vi "TEST - Reorder Array.vi"(8 "error in (no error)":errorcluster) -> (0 "error out":errorcluster, 2 "Pass?":bool=TRUE)   [LabVIEW 2020]
doc: "This VI template can be used for the functional testing of VIs; this implementation includes handling for the testing of polymorphic VIs, and the polymorphic elements should be removed if not needed.\n\nCoded by Douglas A. Femec, January 24, 2006.\n\nCopyright (c) 2005-2006 MKS Instruments, Inc.\nAll rights reserved."
uses:
  TEST - Reorder Array - Inputs.ctl
  Polymorphizer+ Data Type.ctl
  TEST - Reorder Array - Outputs.ctl
  source/library/Reorder Array/Reorder 2D Array (EXT).vi
  source/library/Reorder Array/Reorder 1D Array (EXT).vi
  source/library/Reorder Array/Reorder 2D Array (Boolean).vi
  source/library/Reorder Array/Reorder 1D Array (Boolean).vi
  source/library/Reorder Array/Reorder 2D Array (Variant).vi
  source/library/Reorder Array/Reorder 1D Array (Variant).vi
  source/library/Reorder Array/Reorder 2D Array (DBL).vi
  source/library/Reorder Array/Reorder 1D Array (DBL).vi
  source/library/Reorder Array/Reorder 2D Array (SGL).vi
  source/library/Reorder Array/Reorder 1D Array (SGL).vi
  source/library/Reorder Array/Reorder 2D Array (I32).vi
  source/library/Reorder Array/Reorder 1D Array (I32).vi
  source/library/Reorder Array/Reorder 2D Array (I16).vi
  source/library/Reorder Array/Reorder 1D Array (I16).vi
  source/library/Reorder Array/Reorder 2D Array (I8).vi
  source/library/Reorder Array/Reorder 1D Array (I8).vi
  source/library/Reorder Array/Reorder 2D Array (U32).vi
  source/library/Reorder Array/Reorder 1D Array (U32).vi
  source/library/Reorder Array/Reorder 2D Array (U16).vi
  source/library/Reorder Array/Reorder 1D Array (U16).vi
  source/library/Reorder Array/Reorder 2D Array (U8).vi
  source/library/Reorder Array/Reorder 1D Array (U8).vi
  source/library/Reorder Array/Reorder 2D Array (CXT).vi
  source/library/Reorder Array/Reorder 1D Array (CXT).vi
  source/library/Reorder Array/Reorder 2D Array (CDB).vi
  source/library/Reorder Array/Reorder 1D Array (CDB).vi
  source/library/Reorder Array/Reorder 2D Array (CSG).vi
  source/library/Reorder Array/Reorder 1D Array (CSG).vi
  source/library/Reorder Array/Reorder 2D Array (String).vi
  source/library/Reorder Array/Reorder 1D Array (String).vi
  source/library/Reorder Array/Reorder 2D Array (Path).vi
  source/library/Reorder Array/Reorder 1D Array (Path).vi
  source/library/openg_array.lvlib
panel:
  out "Generated Outputs":T1[][](array[typedef]) {"1D Array" format="%.2f"; "2D Array" format="%.2f"}
  in  "Expected Outputs":T1[](array[typedef])=[{"Description"="Expect empty arrays", "1D Array"=[], "2D Array"=[], "1D Sorted Pointers"=[], "2D Sorted Pointer"=[], "Sort By in"=enum."row"}, {"Description"="Expect empty arrays", "1D Array"=[], "2D Array"=[], "1D Sorted Pointers"=[], "2D Sorted Pointer"=[], "Sort By in"=enum."row"}, {"Description"="Expect empty arrays", "1D Array"=[], "2D Array"=[], "1D Sorted Pointers"=[], "2D Sorted Pointer"=[], "Sort By in"=enum."row"}, {"Description"="Expect empty arrays", "1D Array"=[], "2D Array"=[], "1D Sorted Pointers"=[], "2D Sorted Pointer"=[], "Sort By in"=enum."column"}, {"Description"="Expect empty arrays", "1D Array"=[], "2D Array"=[], "1D Sorted Pointers"=[], "2D Sorted Pointer"=[], "Sort By in"=enum."column"}, {"Description"="Expect empty arrays", "1D Array"=[], "2D Array"=[], "1D Sorted Pointers"=[], "2D Sorted Pointer"=[], "Sort By in"=enum."column"}, {"Description"="Expect empty arrays", "1D Array"=[], "2D Array"=[], "1D Sorted Pointers"=[], "2D Sorted Pointer"=[], "Sort By in"=enum."row"}, {"Description"="Expect empty arrays", "1D Array"=[], "2D Array"=[], "1D Sorted Pointers"=[], "2D Sorted Pointer"=[], "Sort By in"=enum."row"}, {"Description"="Expect empty arrays", "1D Array"=[], "2D Array"=[], "1D Sorted Pointers"=[], "2D Sorted Pointer"=[], "Sort By in"=enum."row"}, {"Description"="Expect empty arrays", "1D Array"=[], "2D Array"=[], "1D Sorted Pointers"=[], "2D Sorted Pointer"=[], "Sort By in"=enum."column"}, {"Description"="Expect empty arrays", "1D Array"=[], "2D Array"=[], "1D Sorted Pointers"=[], "2D Sorted Pointer"=[], "Sort By in"=enum."column"}, {"Description"="Expect empty arrays", "1D Array"=[], "2D Array"=[], "1D Sorted Pointers"=[], "2D Sorted Pointer"=[], "Sort By in"=enum."column"}, {"Description"="Expect sorted in ascending order, 2D by row 0", "1D Array"=[0.0, 1.0, 2.0, 3.0, 4.0], "2D Array"=[[0.0, 5.0], [1.0, 6.0], [2.0, 7.0], [3.0, 8.0], [4.0, 9.0]], "1D Sorted Pointers"=[0, 1, 2, 3, 4], "2D Sorted Pointer"=[0, 1], "Sort By in"=enum."row"}, {"Description"="Expect sorted in ascending order, 2D by row 1", "1D Array"=[0.0, 1.0, 2.0, 3.0, 4.0], "2D Array"=[[0.0, 5.0], [1.0, 6.0], [2.0, 7.0], [3.0, 8.0], [4.0, 9.0]], "1D Sorted Pointers"=[0, 1, 2, 3, 4], "2D Sorted Pointer"=[0, 1], "Sort By in"=enum."row"}, {"Description"="Expect sorted in ascending order, 2D no row 5, so expect index out of range", "1D Array"=[0.0, 1.0, 2.0, 3.0, 4.0], "2D Array"=[], "1D Sorted Pointers"=[0, 1, 2, 3, 4], "2D Sorted Pointer"=[], "Sort By in"=enum."row"}, {"Description"="Expect sorted in ascending order, 2D by column 0", "1D Array"=[0.0, 1.0, 2.0, 3.0, 4.0], "2D Array"=[[0.0, 5.0], [1.0, 6.0], [2.0, 7.0], [3.0, 8.0], [4.0, 9.0]], "1D Sorted Pointers"=[0, 1, 2, 3, 4], "2D Sorted Pointer"=[0, 1, 2, 3, 4], "Sort By in"=enum."column"}, {"Description"="Expect sorted in ascending order, 2D by column 1", "1D Array"=[0.0, 1.0, 2.0, 3.0, 4.0], "2D Array"=[[0.0, 5.0], [1.0, 6.0], [2.0, 7.0], [3.0, 8.0], [4.0, 9.0]], "1D Sorted Pointers"=[0, 1, 2, 3, 4], "2D Sorted Pointer"=[0, 1, 2, 3, 4], "Sort By in"=enum."column"}, {"Description"="Expect sorted in ascending order, 2D no column 5, so expect index out of range", "1D Array"=[0.0, 1.0, 2.0, 3.0, 4.0], "2D Array"=[], "1D Sorted Pointers"=[0, 1, 2, 3, 4], "2D Sorted Pointer"=[], "Sort By in"=enum."column"}, {"Description"="Expect sorted in descending order, 2D by row 0", "1D Array"=[4.0, 3.0, 2.0, 1.0, 0.0], "2D Array"=[[5.0, 0.0], [6.0, 1.0], [7.0, 2.0], [8.0, 3.0], [9.0, 4.0]], "1D Sorted Pointers"=[4, 3, 2, 1, 0], "2D Sorted Pointer"=[1, 0], "Sort By in"=enum."row"}, {"Description"="Expect sorted in descending order, 2D by row 1", "1D Array"=[4.0, 3.0, 2.0, 1.0, 0.0], "2D Array"=[[5.0, 0.0], [6.0, 1.0], [7.0, 2.0], [8.0, 3.0], [9.0, 4.0]], "1D Sorted Pointers"=[4, 3, 2, 1, 0], "2D Sorted Pointer"=[1, 0], "Sort By in"=enum."row"}, {"Description"="Expect sorted in descending order, 2D no row 5, so expect index out of range", "1D Array"=[4.0, 3.0, 2.0, 1.0, 0.0], "2D Array"=[], "1D Sorted Pointers"=[4, 3, 2, 1, 0], "2D Sorted Pointer"=[], "Sort By in"=enum."row"}, {"Description"="Expect sorted in descending order, 2D by column 0", "1D Array"=[4.0, 3.0, 2.0, 1.0, 0.0], "2D Array"=[[4.0, 9.0], [3.0, 8.0], [2.0, 7.0], [1.0, 6.0], [0.0, 5.0]], "1D Sorted Pointers"=[4, 3, 2, 1, 0], "2D Sorted Pointer"=[4, 3, 2, 1, 0], "Sort By in"=enum."column"}, {"Description"="Expect sorted in descending order, 2D by column 1", "1D Array"=[4.0, 3.0, 2.0, 1.0, 0.0], "2D Array"=[[4.0, 9.0], [3.0, 8.0], [2.0, 7.0], [1.0, 6.0], [0.0, 5.0]], "1D Sorted Pointers"=[4, 3, 2, 1, 0], "2D Sorted Pointer"=[4, 3, 2, 1, 0], "Sort By in"=enum."column"}, {"Description"="Expect sorted in descending order, 2D no column 5, so expect index out of range", "1D Array"=[4.0, 3.0, 2.0, 1.0, 0.0], "2D Array"=[], "1D Sorted Pointers"=[4, 3, 2, 1, 0], "2D Sorted Pointer"=[], "Sort By in"=enum."column"}, {"Description"="Expect sorted in ascending order, 2D by row 0", "1D Array"=[0.0, 1.0, 2.0, 3.0, 4.0], "2D Array"=[[4.0, 9.0], [3.0, 8.0], [2.0, 7.0], [1.0, 6.0], [0.0, 5.0]], "1D Sorted Pointers"=[4, 3, 2, 1, 0], "2D Sorted Pointer"=[1, 0], "Sort By in"=enum."row"}, {"Description"="Expect sorted in ascending order, 2D by row 1", "1D Array"=[0.0, 1.0, 2.0, 3.0, 4.0], "2D Array"=[[4.0, 9.0], [3.0, 8.0], [2.0, 7.0], [1.0, 6.0], [0.0, 5.0]], "1D Sorted Pointers"=[4, 3, 2, 1, 0], "2D Sorted Pointer"=[1, 0], "Sort By in"=enum."row"}, {"Description"="Expect sorted in ascending order, 2D no row 5, so expect index out of range", "1D Array"=[0.0, 1.0, 2.0, 3.0, 4.0], "2D Array"=[], "1D Sorted Pointers"=[4, 3, 2, 1, 0], "2D Sorted Pointer"=[], "Sort By in"=enum."row"}, {"Description"="Expect sorted in descending order, 2D by column 0", "1D Array"=[0.0, 1.0, 2.0, 3.0, 4.0], "2D Array"=[[5.0, 0.0], [6.0, 1.0], [7.0, 2.0], [8.0, 3.0], [9.0, 4.0]], "1D Sorted Pointers"=[4, 3, 2, 1, 0], "2D Sorted Pointer"=[4, 3, 2, 1, 0], "Sort By in"=enum."column"}, {"Description"="Expect sorted in descending order, 2D by column 1", "1D Array"=[0.0, 1.0, 2.0, 3.0, 4.0], "2D Array"=[[5.0, 0.0], [6.0, 1.0], [7.0, 2.0], [8.0, 3.0], [9.0, 4.0]], "1D Sorted Pointers"=[4, 3, 2, 1, 0], "2D Sorted Pointer"=[4, 3, 2, 1, 0], "Sort By in"=enum."column"}, {"Description"="Expect sorted in descending order, 2D no column 5, so expect index out of range", "1D Array"=[0.0, 1.0, 2.0, 3.0, 4.0], "2D Array"=[], "1D Sorted Pointers"=[4, 3, 2, 1, 0], "2D Sorted Pointer"=[], "Sort By in"=enum."column"}, {"Description"="Expect sorted in descending order, 2D by row 0", "1D Array"=[4.0, 3.0, 2.0, 1.0, 0.0], "2D Array"=[[9.0, 4.0], [8.0, 3.0], [7.0, 2.0], [6.0, 1.0], [5.0, 0.0]], "1D Sorted Pointers"=[0, 1, 2, 3, 4], "2D Sorted Pointer"=[0, 1], "Sort By in"=enum."row"}, {"Description"="Expect sorted in descending order, 2D by row 1", "1D Array"=[4.0, 3.0, 2.0, 1.0, 0.0], "2D Array"=[[9.0, 4.0], [8.0, 3.0], [7.0, 2.0], [6.0, 1.0], [5.0, 0.0]], "1D Sorted Pointers"=[0, 1, 2, 3, 4], "2D Sorted Pointer"=[0, 1], "Sort By in"=enum."row"}, {"Description"="Expect sorted in descending order, 2D no row 5, so expect index out of range", "1D Array"=[4.0, 3.0, 2.0, 1.0, 0.0], "2D Array"=[], "1D Sorted Pointers"=[0, 1, 2, 3, 4], "2D Sorted Pointer"=[], "Sort By in"=enum."row"}, {"Description"="Expect sorted in descending order, 2D by column 0", "1D Array"=[4.0, 3.0, 2.0, 1.0, 0.0], "2D Array"=[[9.0, 4.0], [8.0, 3.0], [7.0, 2.0], [6.0, 1.0], [5.0, 0.0]], "1D Sorted Pointers"=[0, 1, 2, 3, 4], "2D Sorted Pointer"=[0, 1, 2, 3, 4], "Sort By in"=enum."column"}, {"Description"="Expect sorted in descending order, 2D by column 1", "1D Array"=[4.0, 3.0, 2.0, 1.0, 0.0], "2D Array"=[[9.0, 4.0], [8.0, 3.0], [7.0, 2.0], [6.0, 1.0], [5.0, 0.0]], "1D Sorted Pointers"=[0, 1, 2, 3, 4], "2D Sorted Pointer"=[0, 1, 2, 3, 4], "Sort By in"=enum."column"}, {"Description"="Expect sorted in descending order, 2D no column 5, so expect index out of range", "1D Array"=[4.0, 3.0, 2.0, 1.0, 0.0], "2D Array"=[], "1D Sorted Pointers"=[0, 1, 2, 3, 4], "2D Sorted Pointer"=[], "Sort By in"=enum."column"}, {"Description"="Expect sorted in ascending order, 2D by row 0", "1D Array"=[0.0, 1.0, 2.0, 3.0, 4.0], "2D Array"=[[3.0, 6.0], [2.0, 9.0], [0.0, 5.0], [4.0, 7.0], [1.0, 8.0]], "1D Sorted Pointers"=[2, 4, 1, 0, 3], "2D Sorted Pointer"=[0, 1], "Sort By in"=enum."row"}, {"Description"="Expect sorted in ascending order, 2D by row 1", "1D Array"=[0.0, 1.0, 2.0, 3.0, 4.0], "2D Array"=[[3.0, 6.0], [2.0, 9.0], [0.0, 5.0], [4.0, 7.0], [1.0, 8.0]], "1D Sorted Pointers"=[2, 4, 1, 0, 3], "2D Sorted Pointer"=[0, 1], "Sort By in"=enum."row"}, {"Description"="Expect sorted in ascending order, 2D no row 5, so expect index out of range", "1D Array"=[0.0, 1.0, 2.0, 3.0, 4.0], "2D Array"=[], "1D Sorted Pointers"=[2, 4, 1, 0, 3], "2D Sorted Pointer"=[], "Sort By in"=enum."row"}, {"Description"="Expect sorted in ascending order, 2D by column 0", "1D Array"=[0.0, 1.0, 2.0, 3.0, 4.0], "2D Array"=[[0.0, 5.0], [1.0, 8.0], [2.0, 9.0], [3.0, 6.0], [4.0, 7.0]], "1D Sorted Pointers"=[2, 4, 1, 0, 3], "2D Sorted Pointer"=[2, 4, 1, 0, 3], "Sort By in"=enum."column"}, {"Description"="Expect sorted in ascending order, 2D by column 1", "1D Array"=[0.0, 1.0, 2.0, 3.0, 4.0], "2D Array"=[[0.0, 5.0], [3.0, 6.0], [4.0, 7.0], [1.0, 8.0], [2.0, 9.0]], "1D Sorted Pointers"=[2, 4, 1, 0, 3], "2D Sorted Pointer"=[2, 0, 3, 4, 1], "Sort By in"=enum."column"}, {"Description"="Expect sorted in ascending order, 2D no column 5, so expect index out of range", "1D Array"=[0.0, 1.0, 2.0, 3.0, 4.0], "2D Array"=[], "1D Sorted Pointers"=[2, 4, 1, 0, 3], "2D Sorted Pointer"=[], "Sort By in"=enum."column"}, {"Description"="Expect sorted in descending order, 2D by row 0", "1D Array"=[4.0, 3.0, 2.0, 1.0, 0.0], "2D Array"=[[6.0, 3.0], [9.0, 2.0], [5.0, 0.0], [7.0, 4.0], [8.0, 1.0]], "1D Sorted Pointers"=[3, 0, 1, 4, 2], "2D Sorted Pointer"=[1, 0], "Sort By in"=enum."row"}, {"Description"="Expect sorted in descending order, 2D by row 1", "1D Array"=[4.0, 3.0, 2.0, 1.0, 0.0], "2D Array"=[[6.0, 3.0], [9.0, 2.0], [5.0, 0.0], [7.0, 4.0], [8.0, 1.0]], "1D Sorted Pointers"=[3, 0, 1, 4, 2], "2D Sorted Pointer"=[1, 0], "Sort By in"=enum."row"}, {"Description"="Expect sorted in descending order, 2D no row 5, so expect index out of range", "1D Array"=[4.0, 3.0, 2.0, 1.0, 0.0], "2D Array"=[], "1D Sorted Pointers"=[3, 0, 1, 4, 2], "2D Sorted Pointer"=[], "Sort By in"=enum."row"}, {"Description"="Expect sorted in descending order, 2D by column 0", "1D Array"=[4.0, 3.0, 2.0, 1.0, 0.0], "2D Array"=[[4.0, 7.0], [3.0, 6.0], [2.0, 9.0], [1.0, 8.0], [0.0, 5.0]], "1D Sorted Pointers"=[3, 0, 1, 4, 2], "2D Sorted Pointer"=[3, 0, 1, 4, 2], "Sort By in"=enum."column"}, {"Description"="Expect sorted in descending order, 2D by column 1", "1D Array"=[4.0, 3.0, 2.0, 1.0, 0.0], "2D Array"=[[2.0, 9.0], [1.0, 8.0], [4.0, 7.0], [3.0, 6.0], [0.0, 5.0]], "1D Sorted Pointers"=[3, 0, 1, 4, 2], "2D Sorted Pointer"=[1, 4, 3, 0, 2], "Sort By in"=enum."column"}, {"Description"="Expect sorted in ascending order, 2D no column 5, so expect index out of range", "1D Array"=[4.0, 3.0, 2.0, 1.0, 0.0], "2D Array"=[], "1D Sorted Pointers"=[3, 0, 1, 4, 2], "2D Sorted Pointer"=[], "Sort By in"=enum."column"}] {"1D Array" format="%.2f"; "2D Array" format="%.2f"}
  in  "Inputs":T2[](array[typedef])=[{"Description"="Empty arrays, ascending, 2D by row 0", "Data Types to Test"=[enum."EXT", enum."DBL", enum."SGL", enum."I32", enum."I16", enum."I8", enum."U32", enum."U16", enum."U8", enum."CXT", enum."CDB", enum."CSG", enum."String", enum."Path"], "1D Array"=[], "2D Array"=[], "1D Sorted Pointers"=[], "2D Sorted Pointers"=[], "Sort By in"=enum."row"}, {"Description"="Empty arrays, ascending, 2D by row 1", "Data Types to Test"=[enum."EXT", enum."DBL", enum."SGL", enum."I32", enum."I16", enum."I8", enum."U32", enum."U16", enum."U8", enum."CXT", enum."CDB", enum."CSG", enum."String", enum."Path"], "1D Array"=[], "2D Array"=[], "1D Sorted Pointers"=[], "2D Sorted Pointers"=[], "Sort By in"=enum."row"}, {"Description"="Empty arrays, ascending, 2D by row 5", "Data Types to Test"=[enum."EXT", enum."DBL", enum."SGL", enum."I32", enum."I16", enum."I8", enum."U32", enum."U16", enum."U8", enum."CXT", enum."CDB", enum."CSG", enum."String", enum."Path"], "1D Array"=[], "2D Array"=[], "1D Sorted Pointers"=[], "2D Sorted Pointers"=[], "Sort By in"=enum."row"}, {"Description"="Empty arrays, ascending, 2D by column 0", "Data Types to Test"=[enum."EXT", enum."DBL", enum."SGL", enum."I32", enum."I16", enum."I8", enum."U32", enum."U16", enum."U8", enum."CXT", enum."CDB", enum."CSG", enum."String", enum."Path"], "1D Array"=[], "2D Array"=[], "1D Sorted Pointers"=[], "2D Sorted Pointers"=[], "Sort By in"=enum."column"}, {"Description"="Empty arrays, ascending, 2D by column 1", "Data Types to Test"=[enum."EXT", enum."DBL", enum."SGL", enum."I32", enum."I16", enum."I8", enum."U32", enum."U16", enum."U8", enum."CXT", enum."CDB", enum."CSG", enum."String", enum."Path"], "1D Array"=[], "2D Array"=[], "1D Sorted Pointers"=[], "2D Sorted Pointers"=[], "Sort By in"=enum."column"}, {"Description"="Empty arrays, ascending, 2D by column 5", "Data Types to Test"=[enum."EXT", enum."DBL", enum."SGL", enum."I32", enum."I16", enum."I8", enum."U32", enum."U16", enum."U8", enum."CXT", enum."CDB", enum."CSG", enum."String", enum."Path"], "1D Array"=[], "2D Array"=[], "1D Sorted Pointers"=[], "2D Sorted Pointers"=[], "Sort By in"=enum."column"}, {"Description"="Empty arrays, descending, 2D by row 0", "Data Types to Test"=[enum."EXT", enum."DBL", enum."SGL", enum."I32", enum."I16", enum."I8", enum."U32", enum."U16", enum."U8", enum."CXT", enum."CDB", enum."CSG", enum."String", enum."Path"], "1D Array"=[], "2D Array"=[], "1D Sorted Pointers"=[], "2D Sorted Pointers"=[], "Sort By in"=enum."row"}, {"Description"="Empty arrays, descending, 2D by row 1", "Data Types to Test"=[enum."EXT", enum."DBL", enum."SGL", enum."I32", enum."I16", enum."I8", enum."U32", enum."U16", enum."U8", enum."CXT", enum."CDB", enum."CSG", enum."String", enum."Path"], "1D Array"=[], "2D Array"=[], "1D Sorted Pointers"=[], "2D Sorted Pointers"=[], "Sort By in"=enum."row"}, {"Description"="Empty arrays, descending, 2D by row 5", "Data Types to Test"=[enum."EXT", enum."DBL", enum."SGL", enum."I32", enum."I16", enum."I8", enum."U32", enum."U16", enum."U8", enum."CXT", enum."CDB", enum."CSG", enum."String", enum."Path"], "1D Array"=[], "2D Array"=[], "1D Sorted Pointers"=[], "2D Sorted Pointers"=[], "Sort By in"=enum."row"}, {"Description"="Empty arrays, descending, 2D by column 0", "Data Types to Test"=[enum."EXT", enum."DBL", enum."SGL", enum."I32", enum."I16", enum."I8", enum."U32", enum."U16", enum."U8", enum."CXT", enum."CDB", enum."CSG", enum."String", enum."Path"], "1D Array"=[], "2D Array"=[], "1D Sorted Pointers"=[], "2D Sorted Pointers"=[], "Sort By in"=enum."column"}, {"Description"="Empty arrays, descending, 2D by column 1", "Data Types to Test"=[enum."EXT", enum."DBL", enum."SGL", enum."I32", enum."I16", enum."I8", enum."U32", enum."U16", enum."U8", enum."CXT", enum."CDB", enum."CSG", enum."String", enum."Path"], "1D Array"=[], "2D Array"=[], "1D Sorted Pointers"=[], "2D Sorted Pointers"=[], "Sort By in"=enum."column"}, {"Description"="Empty arrays, descending, 2D by column 5", "Data Types to Test"=[enum."EXT", enum."DBL", enum."SGL", enum."I32", enum."I16", enum."I8", enum."U32", enum."U16", enum."U8", enum."CXT", enum."CDB", enum."CSG", enum."String", enum."Path"], "1D Array"=[], "2D Array"=[], "1D Sorted Pointers"=[], "2D Sorted Pointers"=[], "Sort By in"=enum."column"}, {"Description"="Already sorted in ascending order, ascending, 2D by row 0", "Data Types to Test"=[enum."EXT", enum."DBL", enum."SGL", enum."I32", enum."I16", enum."I8", enum."U32", enum."U16", enum."U8", enum."CXT", enum."CDB", enum."CSG", enum."String", enum."Path"], "1D Array"=[0.0, 1.0, 2.0, 3.0, 4.0], "2D Array"=[[0.0, 5.0], [1.0, 6.0], [2.0, 7.0], [3.0, 8.0], [4.0, 9.0]], "1D Sorted Pointers"=[0, 1, 2, 3, 4], "2D Sorted Pointers"=[0, 1], "Sort By in"=enum."row"}, {"Description"="Already sorted in ascending order, ascending, 2D by row 1", "Data Types to Test"=[enum."EXT", enum."DBL", enum."SGL", enum."I32", enum."I16", enum."I8", enum."U32", enum."U16", enum."U8", enum."CXT", enum."CDB", enum."CSG", enum."String", enum."Path"], "1D Array"=[0.0, 1.0, 2.0, 3.0, 4.0], "2D Array"=[[0.0, 5.0], [1.0, 6.0], [2.0, 7.0], [3.0, 8.0], [4.0, 9.0]], "1D Sorted Pointers"=[0, 1, 2, 3, 4], "2D Sorted Pointers"=[0, 1], "Sort By in"=enum."row"}, {"Description"="Already sorted in ascending order, ascending, 2D by row 5", "Data Types to Test"=[enum."EXT", enum."DBL", enum."SGL", enum."I32", enum."I16", enum."I8", enum."U32", enum."U16", enum."U8", enum."CXT", enum."CDB", enum."CSG", enum."String", enum."Path"], "1D Array"=[0.0, 1.0, 2.0, 3.0, 4.0], "2D Array"=[], "1D Sorted Pointers"=[0, 1, 2, 3, 4], "2D Sorted Pointers"=[], "Sort By in"=enum."row"}, {"Description"="Already sorted in ascending order, ascending, 2D by column 0", "Data Types to Test"=[enum."EXT", enum."DBL", enum."SGL", enum."I32", enum."I16", enum."I8", enum."U32", enum."U16", enum."U8", enum."CXT", enum."CDB", enum."CSG", enum."String", enum."Path"], "1D Array"=[0.0, 1.0, 2.0, 3.0, 4.0], "2D Array"=[[0.0, 5.0], [1.0, 6.0], [2.0, 7.0], [3.0, 8.0], [4.0, 9.0]], "1D Sorted Pointers"=[0, 1, 2, 3, 4], "2D Sorted Pointers"=[0, 1, 2, 3, 4], "Sort By in"=enum."column"}, {"Description"="Already sorted in ascending order, ascending, 2D by column 1", "Data Types to Test"=[enum."EXT", enum."DBL", enum."SGL", enum."I32", enum."I16", enum."I8", enum."U32", enum."U16", enum."U8", enum."CXT", enum."CDB", enum."CSG", enum."String", enum."Path"], "1D Array"=[0.0, 1.0, 2.0, 3.0, 4.0], "2D Array"=[[0.0, 5.0], [1.0, 6.0], [2.0, 7.0], [3.0, 8.0], [4.0, 9.0]], "1D Sorted Pointers"=[0, 1, 2, 3, 4], "2D Sorted Pointers"=[0, 1, 2, 3, 4], "Sort By in"=enum."column"}, {"Description"="Already sorted in ascending order, ascending, 2D by column 5", "Data Types to Test"=[enum."EXT", enum."DBL", enum."SGL", enum."I32", enum."I16", enum."I8", enum."U32", enum."U16", enum."U8", enum."CXT", enum."CDB", enum."CSG", enum."String", enum."Path"], "1D Array"=[0.0, 1.0, 2.0, 3.0, 4.0], "2D Array"=[], "1D Sorted Pointers"=[0, 1, 2, 3, 4], "2D Sorted Pointers"=[], "Sort By in"=enum."column"}, {"Description"="Already sorted in ascending order, descending, 2D by row 0", "Data Types to Test"=[enum."EXT", enum."DBL", enum."SGL", enum."I32", enum."I16", enum."I8", enum."U32", enum."U16", enum."U8", enum."CXT", enum."CDB", enum."CSG", enum."String", enum."Path"], "1D Array"=[0.0, 1.0, 2.0, 3.0, 4.0], "2D Array"=[[0.0, 5.0], [1.0, 6.0], [2.0, 7.0], [3.0, 8.0], [4.0, 9.0]], "1D Sorted Pointers"=[4, 3, 2, 1, 0], "2D Sorted Pointers"=[1, 0], "Sort By in"=enum."row"}, {"Description"="Already sorted in ascending order, descending, 2D by row 1", "Data Types to Test"=[enum."EXT", enum."DBL", enum."SGL", enum."I32", enum."I16", enum."I8", enum."U32", enum."U16", enum."U8", enum."CXT", enum."CDB", enum."CSG", enum."String", enum."Path"], "1D Array"=[0.0, 1.0, 2.0, 3.0, 4.0], "2D Array"=[[0.0, 5.0], [1.0, 6.0], [2.0, 7.0], [3.0, 8.0], [4.0, 9.0]], "1D Sorted Pointers"=[4, 3, 2, 1, 0], "2D Sorted Pointers"=[1, 0], "Sort By in"=enum."row"}, {"Description"="Already sorted in ascending order, descending, 2D by row 5", "Data Types to Test"=[enum."EXT", enum."DBL", enum."SGL", enum."I32", enum."I16", enum."I8", enum."U32", enum."U16", enum."U8", enum."CXT", enum."CDB", enum."CSG", enum."String", enum."Path"], "1D Array"=[0.0, 1.0, 2.0, 3.0, 4.0], "2D Array"=[], "1D Sorted Pointers"=[4, 3, 2, 1, 0], "2D Sorted Pointers"=[], "Sort By in"=enum."row"}, {"Description"="Already sorted in ascending order, descending, 2D by column 0", "Data Types to Test"=[enum."EXT", enum."DBL", enum."SGL", enum."I32", enum."I16", enum."I8", enum."U32", enum."U16", enum."U8", enum."CXT", enum."CDB", enum."CSG", enum."String", enum."Path"], "1D Array"=[0.0, 1.0, 2.0, 3.0, 4.0], "2D Array"=[[0.0, 5.0], [1.0, 6.0], [2.0, 7.0], [3.0, 8.0], [4.0, 9.0]], "1D Sorted Pointers"=[4, 3, 2, 1, 0], "2D Sorted Pointers"=[4, 3, 2, 1, 0], "Sort By in"=enum."column"}, {"Description"="Already sorted in ascending order, descending, 2D by column 1", "Data Types to Test"=[enum."EXT", enum."DBL", enum."SGL", enum."I32", enum."I16", enum."I8", enum."U32", enum."U16", enum."U8", enum."CXT", enum."CDB", enum."CSG", enum."String", enum."Path"], "1D Array"=[0.0, 1.0, 2.0, 3.0, 4.0], "2D Array"=[[0.0, 5.0], [1.0, 6.0], [2.0, 7.0], [3.0, 8.0], [4.0, 9.0]], "1D Sorted Pointers"=[4, 3, 2, 1, 0], "2D Sorted Pointers"=[4, 3, 2, 1, 0], "Sort By in"=enum."column"}, {"Description"="Already sorted in ascending order, descending, 2D by column 5", "Data Types to Test"=[enum."EXT", enum."DBL", enum."SGL", enum."I32", enum."I16", enum."I8", enum."U32", enum."U16", enum."U8", enum."CXT", enum."CDB", enum."CSG", enum."String", enum."Path"], "1D Array"=[0.0, 1.0, 2.0, 3.0, 4.0], "2D Array"=[], "1D Sorted Pointers"=[4, 3, 2, 1, 0], "2D Sorted Pointers"=[], "Sort By in"=enum."column"}, {"Description"="Already sorted in descending order, ascending, 2D by row 0", "Data Types to Test"=[enum."EXT", enum."DBL", enum."SGL", enum."I32", enum."I16", enum."I8", enum."U32", enum."U16", enum."U8", enum."CXT", enum."CDB", enum."CSG", enum."String", enum."Path"], "1D Array"=[4.0, 3.0, 2.0, 1.0, 0.0], "2D Array"=[[9.0, 4.0], [8.0, 3.0], [7.0, 2.0], [6.0, 1.0], [5.0, 0.0]], "1D Sorted Pointers"=[4, 3, 2, 1, 0], "2D Sorted Pointers"=[1, 0], "Sort By in"=enum."row"}, {"Description"="Already sorted in descending order, ascending, 2D by row 1", "Data Types to Test"=[enum."EXT", enum."DBL", enum."SGL", enum."I32", enum."I16", enum."I8", enum."U32", enum."U16", enum."U8", enum."CXT", enum."CDB", enum."CSG", enum."String", enum."Path"], "1D Array"=[4.0, 3.0, 2.0, 1.0, 0.0], "2D Array"=[[9.0, 4.0], [8.0, 3.0], [7.0, 2.0], [6.0, 1.0], [5.0, 0.0]], "1D Sorted Pointers"=[4, 3, 2, 1, 0], "2D Sorted Pointers"=[1, 0], "Sort By in"=enum."row"}, {"Description"="Already sorted in descending order, ascending, 2D by row 5", "Data Types to Test"=[enum."EXT", enum."DBL", enum."SGL", enum."I32", enum."I16", enum."I8", enum."U32", enum."U16", enum."U8", enum."CXT", enum."CDB", enum."CSG", enum."String", enum."Path"], "1D Array"=[4.0, 3.0, 2.0, 1.0, 0.0], "2D Array"=[], "1D Sorted Pointers"=[4, 3, 2, 1, 0], "2D Sorted Pointers"=[], "Sort By in"=enum."row"}, {"Description"="Already sorted in descending order, ascending, 2D by column 0", "Data Types to Test"=[enum."EXT", enum."DBL", enum."SGL", enum."I32", enum."I16", enum."I8", enum."U32", enum."U16", enum."U8", enum."CXT", enum."CDB", enum."CSG", enum."String", enum."Path"], "1D Array"=[4.0, 3.0, 2.0, 1.0, 0.0], "2D Array"=[[9.0, 4.0], [8.0, 3.0], [7.0, 2.0], [6.0, 1.0], [5.0, 0.0]], "1D Sorted Pointers"=[4, 3, 2, 1, 0], "2D Sorted Pointers"=[4, 3, 2, 1, 0], "Sort By in"=enum."column"}, {"Description"="Already sorted in descending order, ascending, 2D by column 1", "Data Types to Test"=[enum."EXT", enum."DBL", enum."SGL", enum."I32", enum."I16", enum."I8", enum."U32", enum."U16", enum."U8", enum."CXT", enum."CDB", enum."CSG", enum."String", enum."Path"], "1D Array"=[4.0, 3.0, 2.0, 1.0, 0.0], "2D Array"=[[9.0, 4.0], [8.0, 3.0], [7.0, 2.0], [6.0, 1.0], [5.0, 0.0]], "1D Sorted Pointers"=[4, 3, 2, 1, 0], "2D Sorted Pointers"=[4, 3, 2, 1, 0], "Sort By in"=enum."column"}, {"Description"="Already sorted in descending order, ascending, 2D by column 5", "Data Types to Test"=[enum."EXT", enum."DBL", enum."SGL", enum."I32", enum."I16", enum."I8", enum."U32", enum."U16", enum."U8", enum."CXT", enum."CDB", enum."CSG", enum."String", enum."Path"], "1D Array"=[4.0, 3.0, 2.0, 1.0, 0.0], "2D Array"=[], "1D Sorted Pointers"=[4, 3, 2, 1, 0], "2D Sorted Pointers"=[], "Sort By in"=enum."column"}, {"Description"="Already sorted in descending order, descending, 2D by row 0", "Data Types to Test"=[enum."EXT", enum."DBL", enum."SGL", enum."I32", enum."I16", enum."I8", enum."U32", enum."U16", enum."U8", enum."CXT", enum."CDB", enum."CSG", enum."String", enum."Path"], "1D Array"=[4.0, 3.0, 2.0, 1.0, 0.0], "2D Array"=[[9.0, 4.0], [8.0, 3.0], [7.0, 2.0], [6.0, 1.0], [5.0, 0.0]], "1D Sorted Pointers"=[0, 1, 2, 3, 4], "2D Sorted Pointers"=[0, 1], "Sort By in"=enum."row"}, {"Description"="Already sorted in descending order, descending, 2D by row 1", "Data Types to Test"=[enum."EXT", enum."DBL", enum."SGL", enum."I32", enum."I16", enum."I8", enum."U32", enum."U16", enum."U8", enum."CXT", enum."CDB", enum."CSG", enum."String", enum."Path"], "1D Array"=[4.0, 3.0, 2.0, 1.0, 0.0], "2D Array"=[[9.0, 4.0], [8.0, 3.0], [7.0, 2.0], [6.0, 1.0], [5.0, 0.0]], "1D Sorted Pointers"=[0, 1, 2, 3, 4], "2D Sorted Pointers"=[0, 1], "Sort By in"=enum."row"}, {"Description"="Already sorted in descending order, descending, 2D by row 5", "Data Types to Test"=[enum."EXT", enum."DBL", enum."SGL", enum."I32", enum."I16", enum."I8", enum."U32", enum."U16", enum."U8", enum."CXT", enum."CDB", enum."CSG", enum."String", enum."Path"], "1D Array"=[4.0, 3.0, 2.0, 1.0, 0.0], "2D Array"=[], "1D Sorted Pointers"=[0, 1, 2, 3, 4], "2D Sorted Pointers"=[], "Sort By in"=enum."row"}, {"Description"="Already sorted in descending order, descending, 2D by column 0", "Data Types to Test"=[enum."EXT", enum."DBL", enum."SGL", enum."I32", enum."I16", enum."I8", enum."U32", enum."U16", enum."U8", enum."CXT", enum."CDB", enum."CSG", enum."String", enum."Path"], "1D Array"=[4.0, 3.0, 2.0, 1.0, 0.0], "2D Array"=[[9.0, 4.0], [8.0, 3.0], [7.0, 2.0], [6.0, 1.0], [5.0, 0.0]], "1D Sorted Pointers"=[0, 1, 2, 3, 4], "2D Sorted Pointers"=[0, 1, 2, 3, 4], "Sort By in"=enum."column"}, {"Description"="Already sorted in descending order, descending, 2D by column 1", "Data Types to Test"=[enum."EXT", enum."DBL", enum."SGL", enum."I32", enum."I16", enum."I8", enum."U32", enum."U16", enum."U8", enum."CXT", enum."CDB", enum."CSG", enum."String", enum."Path"], "1D Array"=[4.0, 3.0, 2.0, 1.0, 0.0], "2D Array"=[[9.0, 4.0], [8.0, 3.0], [7.0, 2.0], [6.0, 1.0], [5.0, 0.0]], "1D Sorted Pointers"=[0, 1, 2, 3, 4], "2D Sorted Pointers"=[0, 1, 2, 3, 4], "Sort By in"=enum."column"}, {"Description"="Already sorted in descending order, descending, 2D by column 5", "Data Types to Test"=[enum."EXT", enum."DBL", enum."SGL", enum."I32", enum."I16", enum."I8", enum."U32", enum."U16", enum."U8", enum."CXT", enum."CDB", enum."CSG", enum."String", enum."Path"], "1D Array"=[4.0, 3.0, 2.0, 1.0, 0.0], "2D Array"=[], "1D Sorted Pointers"=[0, 1, 2, 3, 4], "2D Sorted Pointers"=[], "Sort By in"=enum."column"}, {"Description"="Not sorted, ascending, 2D by row 0", "Data Types to Test"=[enum."EXT", enum."DBL", enum."SGL", enum."I32", enum."I16", enum."I8", enum."U32", enum."U16", enum."U8", enum."CXT", enum."CDB", enum."CSG", enum."String", enum."Path"], "1D Array"=[3.0, 2.0, 0.0, 4.0, 1.0], "2D Array"=[[3.0, 6.0], [2.0, 9.0], [0.0, 5.0], [4.0, 7.0], [1.0, 8.0]], "1D Sorted Pointers"=[2, 4, 1, 0, 3], "2D Sorted Pointers"=[0, 1], "Sort By in"=enum."row"}, {"Description"="Not sorted, ascending, 2D by row 1", "Data Types to Test"=[enum."EXT", enum."DBL", enum."SGL", enum."I32", enum."I16", enum."I8", enum."U32", enum."U16", enum."U8", enum."CXT", enum."CDB", enum."CSG", enum."String", enum."Path"], "1D Array"=[3.0, 2.0, 0.0, 4.0, 1.0], "2D Array"=[[3.0, 6.0], [2.0, 9.0], [0.0, 5.0], [4.0, 7.0], [1.0, 8.0]], "1D Sorted Pointers"=[2, 4, 1, 0, 3], "2D Sorted Pointers"=[0, 1], "Sort By in"=enum."row"}, {"Description"="Not sorted, ascending, 2D by row 5", "Data Types to Test"=[enum."EXT", enum."DBL", enum."SGL", enum."I32", enum."I16", enum."I8", enum."U32", enum."U16", enum."U8", enum."CXT", enum."CDB", enum."CSG", enum."String", enum."Path"], "1D Array"=[3.0, 2.0, 0.0, 4.0, 1.0], "2D Array"=[], "1D Sorted Pointers"=[2, 4, 1, 0, 3], "2D Sorted Pointers"=[], "Sort By in"=enum."row"}, {"Description"="Not sorted, ascending, 2D by column 0", "Data Types to Test"=[enum."EXT", enum."DBL", enum."SGL", enum."I32", enum."I16", enum."I8", enum."U32", enum."U16", enum."U8", enum."CXT", enum."CDB", enum."CSG", enum."String", enum."Path"], "1D Array"=[3.0, 2.0, 0.0, 4.0, 1.0], "2D Array"=[[3.0, 6.0], [2.0, 9.0], [0.0, 5.0], [4.0, 7.0], [1.0, 8.0]], "1D Sorted Pointers"=[2, 4, 1, 0, 3], "2D Sorted Pointers"=[2, 4, 1, 0, 3], "Sort By in"=enum."column"}, {"Description"="Not sorted, ascending, 2D by column 1", "Data Types to Test"=[enum."EXT", enum."DBL", enum."SGL", enum."I32", enum."I16", enum."I8", enum."U32", enum."U16", enum."U8", enum."CXT", enum."CDB", enum."CSG", enum."String", enum."Path"], "1D Array"=[3.0, 2.0, 0.0, 4.0, 1.0], "2D Array"=[[3.0, 6.0], [2.0, 9.0], [0.0, 5.0], [4.0, 7.0], [1.0, 8.0]], "1D Sorted Pointers"=[2, 4, 1, 0, 3], "2D Sorted Pointers"=[2, 0, 3, 4, 1], "Sort By in"=enum."column"}, {"Description"="Not sorted, ascending, 2D by column 5", "Data Types to Test"=[enum."EXT", enum."DBL", enum."SGL", enum."I32", enum."I16", enum."I8", enum."U32", enum."U16", enum."U8", enum."CXT", enum."CDB", enum."CSG", enum."String", enum."Path"], "1D Array"=[3.0, 2.0, 0.0, 4.0, 1.0], "2D Array"=[], "1D Sorted Pointers"=[2, 4, 1, 0, 3], "2D Sorted Pointers"=[], "Sort By in"=enum."column"}, {"Description"="Not sorted, descending, 2D by row 0", "Data Types to Test"=[enum."EXT", enum."DBL", enum."SGL", enum."I32", enum."I16", enum."I8", enum."U32", enum."U16", enum."U8", enum."CXT", enum."CDB", enum."CSG", enum."String", enum."Path"], "1D Array"=[3.0, 2.0, 0.0, 4.0, 1.0], "2D Array"=[[3.0, 6.0], [2.0, 9.0], [0.0, 5.0], [4.0, 7.0], [1.0, 8.0]], "1D Sorted Pointers"=[3, 0, 1, 4, 2], "2D Sorted Pointers"=[1, 0], "Sort By in"=enum."row"}, {"Description"="Not sorted, descending, 2D by row 1", "Data Types to Test"=[enum."EXT", enum."DBL", enum."SGL", enum."I32", enum."I16", enum."I8", enum."U32", enum."U16", enum."U8", enum."CXT", enum."CDB", enum."CSG", enum."String", enum."Path"], "1D Array"=[3.0, 2.0, 0.0, 4.0, 1.0], "2D Array"=[[3.0, 6.0], [2.0, 9.0], [0.0, 5.0], [4.0, 7.0], [1.0, 8.0]], "1D Sorted Pointers"=[3, 0, 1, 4, 2], "2D Sorted Pointers"=[1, 0], "Sort By in"=enum."row"}, {"Description"="Not sorted, descending, 2D by row 5", "Data Types to Test"=[enum."EXT", enum."DBL", enum."SGL", enum."I32", enum."I16", enum."I8", enum."U32", enum."U16", enum."U8", enum."CXT", enum."CDB", enum."CSG", enum."String", enum."Path"], "1D Array"=[3.0, 2.0, 0.0, 4.0, 1.0], "2D Array"=[], "1D Sorted Pointers"=[3, 0, 1, 4, 2], "2D Sorted Pointers"=[], "Sort By in"=enum."row"}, {"Description"="Not sorted, descending, 2D by column 0", "Data Types to Test"=[enum."EXT", enum."DBL", enum."SGL", enum."I32", enum."I16", enum."I8", enum."U32", enum."U16", enum."U8", enum."CXT", enum."CDB", enum."CSG", enum."String", enum."Path"], "1D Array"=[3.0, 2.0, 0.0, 4.0, 1.0], "2D Array"=[[3.0, 6.0], [2.0, 9.0], [0.0, 5.0], [4.0, 7.0], [1.0, 8.0]], "1D Sorted Pointers"=[3, 0, 1, 4, 2], "2D Sorted Pointers"=[3, 0, 1, 4, 2], "Sort By in"=enum."column"}, {"Description"="Not sorted, descending, 2D by column 1", "Data Types to Test"=[enum."EXT", enum."DBL", enum."SGL", enum."I32", enum."I16", enum."I8", enum."U32", enum."U16", enum."U8", enum."CXT", enum."CDB", enum."CSG", enum."String", enum."Path"], "1D Array"=[3.0, 2.0, 0.0, 4.0, 1.0], "2D Array"=[[3.0, 6.0], [2.0, 9.0], [0.0, 5.0], [4.0, 7.0], [1.0, 8.0]], "1D Sorted Pointers"=[3, 0, 1, 4, 2], "2D Sorted Pointers"=[1, 4, 3, 0, 2], "Sort By in"=enum."column"}, {"Description"="Not sorted, descending, 2D by column 5", "Data Types to Test"=[enum."EXT", enum."DBL", enum."SGL", enum."I32", enum."I16", enum."I8", enum."U32", enum."U16", enum."U8", enum."CXT", enum."CDB", enum."CSG", enum."String", enum."Path"], "1D Array"=[3.0, 2.0, 0.0, 4.0, 1.0], "2D Array"=[], "1D Sorted Pointers"=[3, 0, 1, 4, 2], "2D Sorted Pointers"=[], "Sort By in"=enum."column"}] {"1D Array" format="%.2f"; "2D Array" format="%.2f"}
  # "Copyright (c) 2005-2006 MKS Instruments, Inc.\nAll rights reserved."
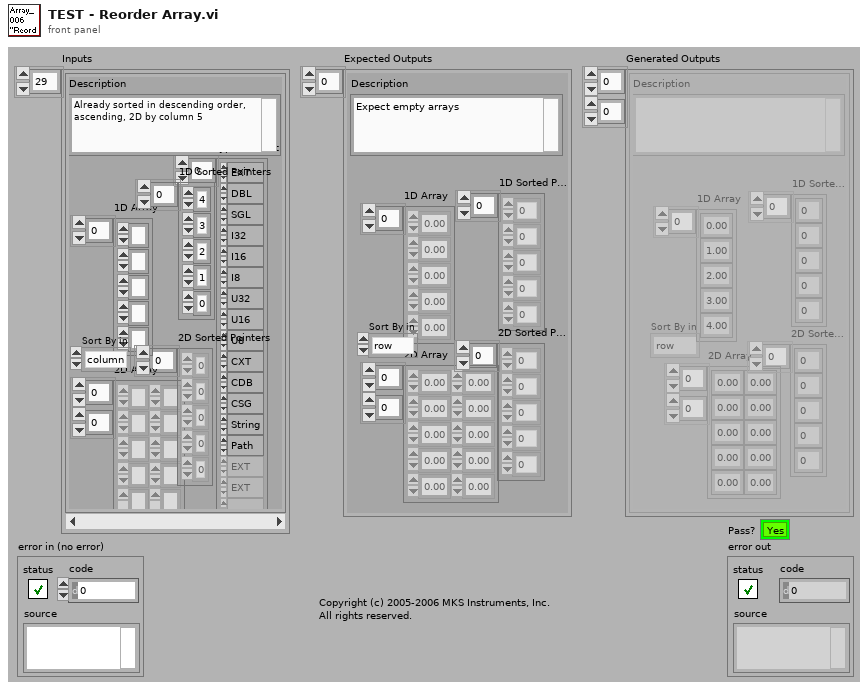
[diagram p1: front panel]
types:
  T1 = typedef "TEST - Reorder Array - Outputs.ctl" = cluster{"Description":string, "1D Array":sgl[], "2D Array":sgl[][], "1D Sorted Pointers":i32[], "2D Sorted Pointer":i32[], "Sort By in":enum16{"row", "column"}}
  T2 = typedef "TEST - Reorder Array - Inputs.ctl" = cluster{"Description":string, "Data Types to Test":T3[], "1D Array":sgl[], "2D Array":sgl[][], "1D Sorted Pointers":i32[], "2D Sorted Pointers":i32[], "Sort By in":enum16{"row", "column"}}
  T3 = typedef "Polymorphizer+ Data Type.ctl" = enum16{"EXT", "DBL", "SGL", "I32", "I16", "I8", "U32", "U16", "U8", "CXT", "CDB", "CSG", "Boolean", "String", "Path", "Variant", "CTL-REF", "GEN-REF", "GObj-REF", "VI-REF", "ENUM", "ERR", "FILE-REF", "MENU-REF", "MENU-RING", "PICT-RING", "TXT&PICT-RING", "TXT-RING", "I64", "U64", "LabVIEW Object"}
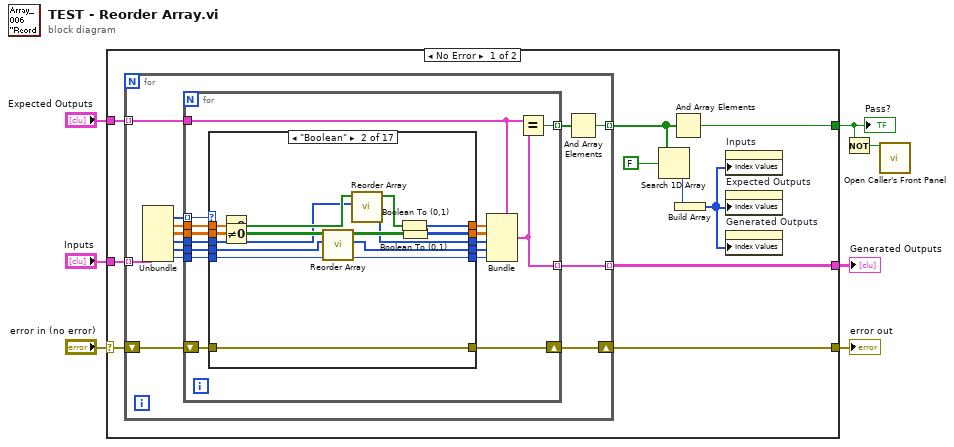
[diagram p0: block diagram]
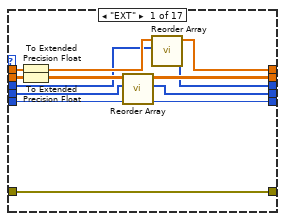
[diagram p2: hidden frame]
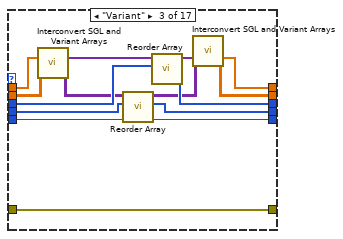
[diagram p3: hidden frame]
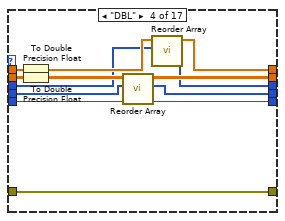
[diagram p4: hidden frame]
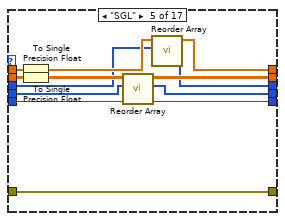
[diagram p5: hidden frame]
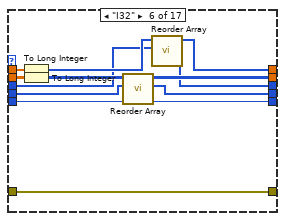
[diagram p6: hidden frame]
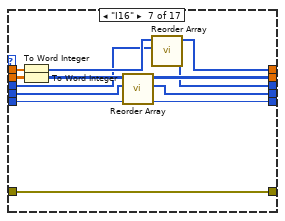
[diagram p7: hidden frame]
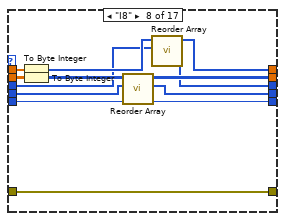
[diagram p8: hidden frame]
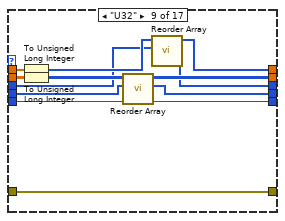
[diagram p9: hidden frame]
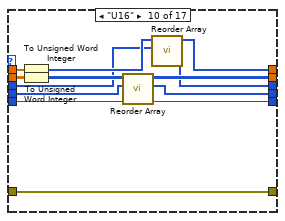
[diagram p10: hidden frame]
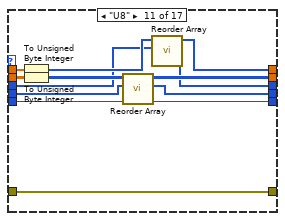
[diagram p11: hidden frame]
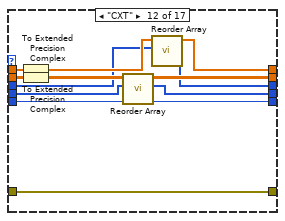
[diagram p12: hidden frame]
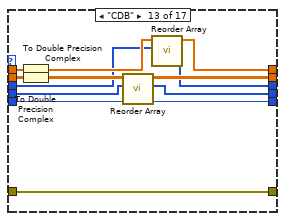
[diagram p13: hidden frame]
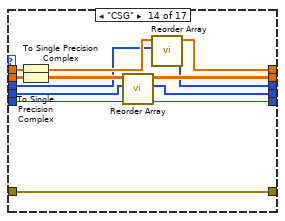
[diagram p14: hidden frame]
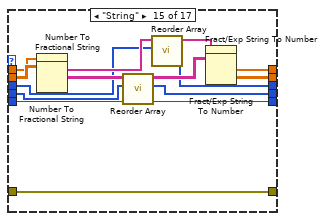
[diagram p15: hidden frame]
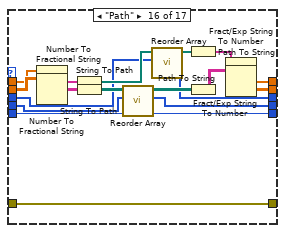
[diagram p16: hidden frame]
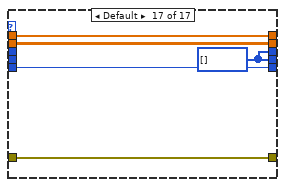
[diagram p17: hidden frame]
diagram:
  n1 = case shown="No Error" "error in (no error)" {
    selector: "error in (no error)" -> [w16 w272]
    tunnel: [w17 w272] -> w6
    tunnel: "Expected Outputs" -> [w14 _]
    tunnel: "Inputs" -> [w15 _]
    tunnel: [w13 _] -> w3
    tunnel: [w12 _] -> w1
    frame No Error {
      n2 = for {
        shift-right: [w25] -> w17
        shift-left: w16 -> [w26]
        tunnel: w15 -> [w27] mode=indexing
        tunnel: w14 -> [w30] mode=indexing
        tunnel: [w29] -> w13 mode=indexing
        tunnel: [w24] -> w11 mode=indexing
        n3 = Unbundle(w27) -> ("Data Types to Test"=w22:T3[], "1D Array"=w20:sgl[], "2D Array"=w21:sgl[][], "1D Sorted Pointers"=w19:i32[], "2D Sorted Pointers"=w18:i32[], "Sort By in"=w23:enum16{"row", "column"})  [unwired: 1 out]
        n4 = for {
          tunnel: w30 -> [w46]
          tunnel: [w44] -> w29 mode=indexing
          tunnel: [w45] -> w28 mode=indexing
          shift-right: [w39] -> w25
          shift-left: w26 -> [w40]
          tunnel: w22 -> [w41] mode=indexing
          tunnel: w20 -> [w43]
          tunnel: w21 -> [w42]
          tunnel: w23 -> [w36]
          tunnel: w19 -> [w35]
          tunnel: w18 -> [w34]
          n5 = case shown="\"Boolean\"" w41 {
            tunnel: w43 -> [w58 w73 w79 w101 w114 w127 w140 w153 w166 w179 w192 w205 w218 w231 w246 w263 w270]
            tunnel: [w55 w61 w77 w98 w111 w124 w137 w150 w163 w176 w189 w202 w215 w228 w240 w256 w270] -> w38
            tunnel: [w54 w60 w75 w97 w110 w123 w136 w149 w162 w175 w188 w201 w214 w227 w239 w257 w269] -> w37
            tunnel: w42 -> [w59 w74 w82 w102 w115 w128 w141 w154 w167 w180 w193 w206 w219 w232 w247 w265 w269]
            tunnel: w40 -> [w56 w71 w89 w99 w112 w125 w138 w151 w164 w177 w190 w203 w216 w229 w245 w262 w271]
            tunnel: [w56 w71 w89 w99 w112 w125 w138 w151 w164 w177 w190 w203 w216 w229 w245 w262 w271] -> w39
            tunnel: w36 -> [w47 w62 w83 w90 w103 w116 w129 w143 w155 w168 w181 w194 w207 w220 w233 w248 w267]
            tunnel: w35 -> [w49 w64 w85 w92 w105 w118 w131 w145 w157 w170 w183 w195 w209 w222 w235 w250 _]
            tunnel: w34 -> [w48 w63 w84 w91 w104 w117 w130 w144 w156 w169 w182 w196 w208 w221 w234 w249 _]
            tunnel: [w51 w66 w87 w94 w107 w120 w133 w146 w159 w172 w185 w198 w212 w224 w237 w252 w268] -> w33
            tunnel: [w52 w67 w88 w95 w108 w121 w134 w147 w160 w173 w186 w199 w211 w225 w238 w253 w268] -> w32
            tunnel: [w50 w65 w86 w93 w106 w119 w132 w142 w158 w171 w184 w197 w210 w223 w236 w251 w267] -> w31
            frame "EXT" {
              n6 = To Extended Precision Float(1:w58) -> (0:w57:ext[])
              n7 = To Extended Precision Float(1:w59) -> (0:w53:ext[][])
              n8 = call-poly "Reorder Array.vi"("Sort By in"=w47, "Sorted Pointers in"=w48, "Array in"=w53) -> ("Sort By out"=w50:enum16{"row", "column"}, "Sorted Pointers out"=w51:i32[], "Sorted Array out"=w54:ext[][])  [unwired: 6 in]
              n9 = call-poly "Reorder Array.vi"("Sorted Pointers in"=w49, "Array in"=w57) -> ("Sorted Pointers out"=w52:i32[], "Sorted Array out"=w55:ext[])  [unwired: 8 in]
            }
            frame "Boolean" {
              n10 = Not Equal To 0?(x=w73) -> (x != 0?=w72:bool[])
              n11 = Not Equal To 0?(x=w74) -> (x != 0?=w68:bool[][])
              n12 = call-poly "Reorder Array.vi"("Sort By in"=w62, "Sorted Pointers in"=w63, "Array in"=w68) -> ("Sort By out"=w65:enum16{"row", "column"}, "Sorted Pointers out"=w66:i32[], "Sorted Array out"=w69:bool[][])  [unwired: 6 in]
              n13 = call-poly "Reorder Array.vi"("Sorted Pointers in"=w64, "Array in"=w72) -> ("Sorted Pointers out"=w67:i32[], "Sorted Array out"=w70:bool[])  [unwired: 8 in]
              n14 = Boolean To (0,1)(Boolean=w70) -> (0, 1=w61:i16[])
              n15 = Boolean To (0,1)(Boolean=w69) -> (0, 1=w60:i16[][])
            }
            frame "Variant" {
              n16 = call "Interconvert SGL and Variant Arrays.vi"("SGL 1D Array 2 In"=w79, "SGL 2D Array In"=w82) -> ("Variant 1D Array 2 Out"=w80:variant[], "Variant 2D Array Out"=w81:variant[][])  [unwired: 9 in, 3 out]
              n17 = call-poly "Reorder Array.vi"("Sort By in"=w83, "Sorted Pointers in"=w84, "Array in"=w81) -> ("Sort By out"=w86:enum16{"row", "column"}, "Sorted Pointers out"=w87:i32[], "Sorted Array out"=w76:variant[][])  [unwired: 6 in]
              n18 = call-poly "Reorder Array.vi"("Sorted Pointers in"=w85, "Array in"=w80) -> ("Sorted Pointers out"=w88:i32[], "Sorted Array out"=w78:variant[])  [unwired: 8 in]
              n19 = call "Interconvert SGL and Variant Arrays.vi"("Variant 1D Array In"=w78, "Variant 2D Array In"=w76) -> ("SGL 1D Array Out"=w77:sgl[], "SGL 2D Array Out"=w75:sgl[][])  [unwired: 9 in, 3 out]
            }
            frame "DBL" {
              n20 = To Double Precision Float(number=w101) -> (double precision float=w100:dbl[])
              n21 = To Double Precision Float(number=w102) -> (double precision float=w96:dbl[][])
              n22 = call-poly "Reorder Array.vi"("Sort By in"=w90, "Sorted Pointers in"=w91, "Array in"=w96) -> ("Sort By out"=w93:enum16{"row", "column"}, "Sorted Pointers out"=w94:i32[], "Sorted Array out"=w97:dbl[][])  [unwired: 6 in]
              n23 = call-poly "Reorder Array.vi"("Sorted Pointers in"=w92, "Array in"=w100) -> ("Sorted Pointers out"=w95:i32[], "Sorted Array out"=w98:dbl[])  [unwired: 8 in]
            }
            frame "SGL" {
              n24 = To Single Precision Float(number=w114) -> (single precision float=w113:sgl[])
              n25 = To Single Precision Float(number=w115) -> (single precision float=w109:sgl[][])
              n26 = call-poly "Reorder Array.vi"("Sort By in"=w103, "Sorted Pointers in"=w104, "Array in"=w109) -> ("Sort By out"=w106:enum16{"row", "column"}, "Sorted Pointers out"=w107:i32[], "Sorted Array out"=w110:sgl[][])  [unwired: 6 in]
              n27 = call-poly "Reorder Array.vi"("Sorted Pointers in"=w105, "Array in"=w113) -> ("Sorted Pointers out"=w108:i32[], "Sorted Array out"=w111:sgl[])  [unwired: 8 in]
            }
            frame "I32" {
              n28 = To Long Integer(number=w127) -> (32bit integer=w126:i32[])
              n29 = To Long Integer(number=w128) -> (32bit integer=w122:i32[][])
              n30 = call-poly "Reorder Array.vi"("Sort By in"=w116, "Sorted Pointers in"=w117, "Array in"=w122) -> ("Sort By out"=w119:enum16{"row", "column"}, "Sorted Pointers out"=w120:i32[], "Sorted Array out"=w123:i32[][])  [unwired: 6 in]
              n31 = call-poly "Reorder Array.vi"("Sorted Pointers in"=w118, "Array in"=w126) -> ("Sorted Pointers out"=w121:i32[], "Sorted Array out"=w124:i32[])  [unwired: 8 in]
            }
            frame "I16" {
              n32 = To Word Integer(number=w140) -> (16bit integer=w139:i16[])
              n33 = To Word Integer(number=w141) -> (16bit integer=w135:i16[][])
              n34 = call-poly "Reorder Array.vi"("Sort By in"=w129, "Sorted Pointers in"=w130, "Array in"=w135) -> ("Sort By out"=w132:enum16{"row", "column"}, "Sorted Pointers out"=w133:i32[], "Sorted Array out"=w136:i16[][])  [unwired: 6 in]
              n35 = call-poly "Reorder Array.vi"("Sorted Pointers in"=w131, "Array in"=w139) -> ("Sorted Pointers out"=w134:i32[], "Sorted Array out"=w137:i16[])  [unwired: 8 in]
            }
            frame "I8" {
              n36 = To Byte Integer(number=w153) -> (8bit integer=w152:i8[])
              n37 = To Byte Integer(number=w154) -> (8bit integer=w148:i8[][])
              n38 = call-poly "Reorder Array.vi"("Sort By in"=w143, "Sorted Pointers in"=w144, "Array in"=w148) -> ("Sort By out"=w142:enum16{"row", "column"}, "Sorted Pointers out"=w146:i32[], "Sorted Array out"=w149:i8[][])  [unwired: 6 in]
              n39 = call-poly "Reorder Array.vi"("Sorted Pointers in"=w145, "Array in"=w152) -> ("Sorted Pointers out"=w147:i32[], "Sorted Array out"=w150:i8[])  [unwired: 8 in]
            }
            frame "U32" {
              n40 = To Unsigned Long Integer(number=w166) -> (unsigned 32bit integer=w165:u32[])
              n41 = To Unsigned Long Integer(number=w167) -> (unsigned 32bit integer=w161:u32[][])
              n42 = call-poly "Reorder Array.vi"("Sort By in"=w155, "Sorted Pointers in"=w156, "Array in"=w161) -> ("Sort By out"=w158:enum16{"row", "column"}, "Sorted Pointers out"=w159:i32[], "Sorted Array out"=w162:u32[][])  [unwired: 6 in]
              n43 = call-poly "Reorder Array.vi"("Sorted Pointers in"=w157, "Array in"=w165) -> ("Sorted Pointers out"=w160:i32[], "Sorted Array out"=w163:u32[])  [unwired: 8 in]
            }
            frame "U16" {
              n44 = To Unsigned Word Integer(number=w179) -> (unsigned 16bit integer=w178:u16[])
              n45 = To Unsigned Word Integer(number=w180) -> (unsigned 16bit integer=w174:u16[][])
              n46 = call-poly "Reorder Array.vi"("Sort By in"=w168, "Sorted Pointers in"=w169, "Array in"=w174) -> ("Sort By out"=w171:enum16{"row", "column"}, "Sorted Pointers out"=w172:i32[], "Sorted Array out"=w175:u16[][])  [unwired: 6 in]
              n47 = call-poly "Reorder Array.vi"("Sorted Pointers in"=w170, "Array in"=w178) -> ("Sorted Pointers out"=w173:i32[], "Sorted Array out"=w176:u16[])  [unwired: 8 in]
            }
            frame "U8" {
              n48 = To Unsigned Byte Integer(number=w192) -> (unsigned 8bit integer=w191:u8[])
              n49 = To Unsigned Byte Integer(number=w193) -> (unsigned 8bit integer=w187:u8[][])
              n50 = call-poly "Reorder Array.vi"("Sort By in"=w181, "Sorted Pointers in"=w182, "Array in"=w187) -> ("Sort By out"=w184:enum16{"row", "column"}, "Sorted Pointers out"=w185:i32[], "Sorted Array out"=w188:u8[][])  [unwired: 6 in]
              n51 = call-poly "Reorder Array.vi"("Sorted Pointers in"=w183, "Array in"=w191) -> ("Sorted Pointers out"=w186:i32[], "Sorted Array out"=w189:u8[])  [unwired: 8 in]
            }
            frame "CXT" {
              n52 = To Extended Precision Complex(1:w205) -> (0:w204:cxt[])
              n53 = To Extended Precision Complex(1:w206) -> (0:w200:cxt[][])
              n54 = call-poly "Reorder Array.vi"("Sort By in"=w194, "Sorted Pointers in"=w196, "Array in"=w200) -> ("Sort By out"=w197:enum16{"row", "column"}, "Sorted Pointers out"=w198:i32[], "Sorted Array out"=w201:cxt[][])  [unwired: 6 in]
              n55 = call-poly "Reorder Array.vi"("Sorted Pointers in"=w195, "Array in"=w204) -> ("Sorted Pointers out"=w199:i32[], "Sorted Array out"=w202:cxt[])  [unwired: 8 in]
            }
            frame "CDB" {
              n56 = To Double Precision Complex(1:w218) -> (0:w217:cdb[])
              n57 = To Double Precision Complex(1:w219) -> (0:w213:cdb[][])
              n58 = call-poly "Reorder Array.vi"("Sort By in"=w207, "Sorted Pointers in"=w208, "Array in"=w213) -> ("Sort By out"=w210:enum16{"row", "column"}, "Sorted Pointers out"=w212:i32[], "Sorted Array out"=w214:cdb[][])  [unwired: 6 in]
              n59 = call-poly "Reorder Array.vi"("Sorted Pointers in"=w209, "Array in"=w217) -> ("Sorted Pointers out"=w211:i32[], "Sorted Array out"=w215:cdb[])  [unwired: 8 in]
            }
            frame "CSG" {
              n60 = To Single Precision Complex(1:w231) -> (0:w230:csg[])
              n61 = To Single Precision Complex(1:w232) -> (0:w226:csg[][])
              n62 = call-poly "Reorder Array.vi"("Sort By in"=w220, "Sorted Pointers in"=w221, "Array in"=w226) -> ("Sort By out"=w223:enum16{"row", "column"}, "Sorted Pointers out"=w224:i32[], "Sorted Array out"=w227:csg[][])  [unwired: 6 in]
              n63 = call-poly "Reorder Array.vi"("Sorted Pointers in"=w222, "Array in"=w230) -> ("Sorted Pointers out"=w225:i32[], "Sorted Array out"=w228:csg[])  [unwired: 8 in]
            }
            frame "String" {
              n64 = Number To Fractional String(number=w246) -> (F-format string=w244:string[])  [unwired: 3 in]
              n65 = Number To Fractional String(number=w247) -> (F-format string=w243:string[][])  [unwired: 3 in]
              n66 = call-poly "Reorder Array.vi"("Sort By in"=w233, "Sorted Pointers in"=w234, "Array in"=w243) -> ("Sort By out"=w236:enum16{"row", "column"}, "Sorted Pointers out"=w237:i32[], "Sorted Array out"=w241:string[][])  [unwired: 6 in]
              n67 = call-poly "Reorder Array.vi"("Sorted Pointers in"=w235, "Array in"=w244) -> ("Sorted Pointers out"=w238:i32[], "Sorted Array out"=w242:string[])  [unwired: 8 in]
              n68 = Fract/Exp String To Number(string=w242) -> (number=w240:dbl[])  [unwired: 3 in, 1 out]
              n69 = Fract/Exp String To Number(string=w241) -> (number=w239:dbl[][])  [unwired: 3 in, 1 out]
            }
            frame "Path" {
              n70 = Number To Fractional String(number=w263) -> (F-format string=w264:string[])  [unwired: 3 in]
              n71 = Number To Fractional String(number=w265) -> (F-format string=w266:string[][])  [unwired: 3 in]
              n72 = String To Path(string=w264) -> (path=w261:path[])
              n73 = String To Path(string=w266) -> (path=w258:path[][])
              n74 = call-poly "Reorder Array.vi"("Sort By in"=w248, "Sorted Pointers in"=w249, "Array in"=w258) -> ("Sort By out"=w251:enum16{"row", "column"}, "Sorted Pointers out"=w252:i32[], "Sorted Array out"=w259:path[][])  [unwired: 6 in]
              n75 = call-poly "Reorder Array.vi"("Sorted Pointers in"=w250, "Array in"=w261) -> ("Sorted Pointers out"=w253:i32[], "Sorted Array out"=w260:path[])  [unwired: 8 in]
              n76 = Path To String(path=w260) -> (string=w255:string[])
              n77 = Path To String(path=w259) -> (string=w254:string[][])
              n78 = Fract/Exp String To Number(string=w255) -> (number=w256:dbl[])  [unwired: 3 in, 1 out]
              n79 = Fract/Exp String To Number(string=w254) -> (number=w257:dbl[][])  [unwired: 3 in, 1 out]
            }
            frame Default {
              w268 = i32[] [] ("Sorted Pointers")
            }
          }
          n80 = Bundle(cluster=w46, "1D Array"=w38, "2D Array"=w37, "1D Sorted Pointers"=w32, "2D Sorted Pointer"=w33, "Sort By in"=w31) -> (w44:T1)  [unwired: 1 in]
          n81 = Equal?(x=w46, y=w44) -> (x = y?=w45:bool)
        }
        n82 = And Array Elements(Boolean array=w28) -> (logical AND=w24:bool)
      }
      n83 = Search 1D Array(1D array=w11, element=FALSE) -> (index of element=w9:i32)  [unwired: 1 in]
      n84 = And Array Elements(Boolean array=w11) -> (logical AND=w12:bool)
      n85 = Build Array(w9) -> (w8:i32[])
      n86 = property on="Inputs" class="Arr (strict)"("Index Values"=w8) -> ()  [unwired: 2 in, 2 out]
      n87 = property on="Expected Outputs" class="Arr (strict)"("Index Values"=w8) -> ()  [unwired: 2 in, 2 out]
      n88 = property on="Generated Outputs" class="Arr (strict)"("Index Values"=w8) -> ()  [unwired: 2 in, 2 out]
    }
    frame Error {
    }
  }
  "error out" <- w6
  "Pass?" <- w1
  "Generated Outputs" <- w3
  n89 = Not(x=w1) -> (.not. x?=w2:bool)
  n90 = call "Open Caller's Front Panel.vi"("Open?"=w2) -> ()  [unwired: 14 in, 1 out]
